vi "test Write and Read Signed Integer Array.vi"(8 "error in (no error)":errorcluster, 11 "TestCase in":refnum<class "Read Value Tests.lvclass">) -> (0 "error out":errorcluster, 3 "TestCase out":refnum<class "Read Value Tests.lvclass">)   [LabVIEW 2017, in "Mem Buff Tests.lvlib" / "Read Value Tests.lvclass"]
uses:
  Read Value Tests.lvclass
  Read Value Tests.lvclass/Read Value Tests.ctl
  Engine/Classes/Buffer/Read 1D I8.vi
  Engine/Classes/Buffer/Read 1D I16.vi
  Engine/Classes/Buffer/Read 1D I32.vi
  Engine/Classes/Buffer/Read 1D I64.vi
  <vilib>/addons/_JKI Toolkits/VI Tester/TestCase.llb/TestCase.lvclass
  Engine/Classes/Buffer/Buffer.lvclass
  C:/Program Files (x86)/National Instruments/LabVIEW 2017/vi.lib/addons/_JKI Toolkits/VI Tester/TestCase.llb/TestCase.lvclass
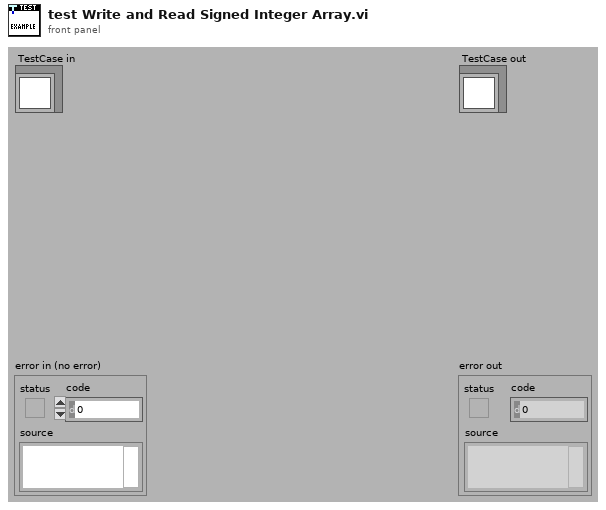
[diagram p1: front panel]
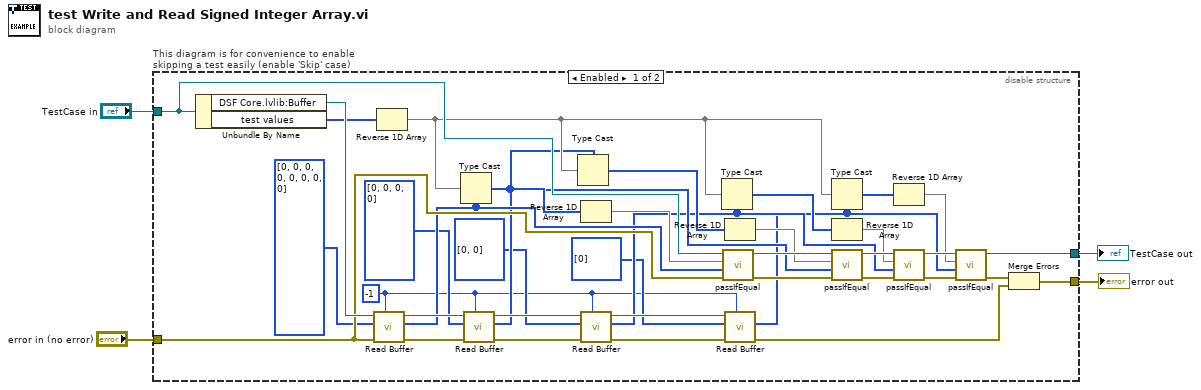
[diagram p0: block diagram]
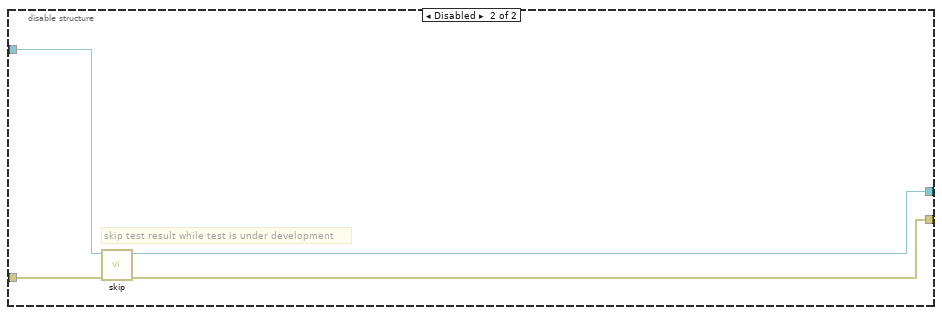
[diagram p2: hidden frame]
diagram:
  n1 = disable-structure "This diagram is for convenience to enable skipping a test easily (enable 'Skip' case)" shown="Enabled" {
    disable-tunnel: "TestCase in" -> [w24 w46]
    disable-tunnel: [w25 w44] -> w1
    disable-tunnel: [w21 w45] -> w2
    disable-tunnel: "error in (no error)" -> [w22 w43]
    frame Enabled {
      w5 = i64 -1 ("count")
      n2 = Unbundle By Name(w24) -> ("DSF Core.lvlib:Buffer"=w23:refnum<class "Buffer.lvclass">, "test values"=w19:u8[])
      n3 = call-poly "Read Buffer.vi"("count"=w5, "error in (no error)"=w22, "buffer in"=i8[] [0, 0, 0, 0, 0, 0, 0, 0], "Buffer in"=w23) -> ("error out"=w41:errorcluster, "buffer out"=w13:i8[], "Buffer out"=w42:refnum<class "Buffer.lvclass">)  [unwired: 4 in, 1 out]
      n4 = Reverse 1D Array(array=w19) -> (reversed array=w18:u8[])
      n5 = Type Cast(type=w13, x=w18) -> (*(type *) &x=w36:i8[])
      n6 = call-poly "Read Buffer.vi"("count"=w5, "error in (no error)"=w41, "buffer in"=i16[] [0, 0, 0, 0], "Buffer in"=w42) -> ("error out"=w39:errorcluster, "buffer out"=w10:i16[], "Buffer out"=w40:refnum<class "Buffer.lvclass">)  [unwired: 4 in, 1 out]
      n7 = Type Cast(type=w10, x=w18) -> (*(type *) &x=w35:i16[])
      n8 = Reverse 1D Array(array=w36) -> (reversed array=w17:i8[])
      n9 = call-poly "Read Buffer.vi"("count"=w5, "error in (no error)"=w39, "buffer in"=i32[] [0, 0], "Buffer in"=w40) -> ("error out"=w37:errorcluster, "buffer out"=w8:i32[], "Buffer out"=w38:refnum<class "Buffer.lvclass">)  [unwired: 4 in, 1 out]
      n10 = Type Cast(type=w8, x=w18) -> (*(type *) &x=w34:i32[])
      n11 = call-dynamic "passIfEqual.vi"("error in (no error)"=w22, "y"=w13, "x"=w17, "TestCase in"=w24) -> ("error out"=w29:errorcluster, "TestCase out"=w30:refnum<class "Read Value Tests.lvclass">)  [unwired: 6 in]
      n12 = Reverse 1D Array(array=w35) -> (reversed array=w16:i16[])
      n13 = call-poly "Read Buffer.vi"("count"=w5, "error in (no error)"=w37, "buffer in"=i64[] [0], "Buffer in"=w38) -> ("error out"=w20:errorcluster, "buffer out"=w6:i64[])  [unwired: 4 in, 2 out]
      n14 = Type Cast(type=w6, x=w18) -> (*(type *) &x=w33:i64[])
      n15 = Reverse 1D Array(array=w34) -> (reversed array=w15:i32[])
      n16 = call-dynamic "passIfEqual.vi"("error in (no error)"=w29, "y"=w10, "x"=w16, "TestCase in"=w30) -> ("error out"=w27:errorcluster, "TestCase out"=w28:refnum<class "Read Value Tests.lvclass">)  [unwired: 6 in]
      n17 = Reverse 1D Array(array=w33) -> (reversed array=w14:i64[])
      n18 = call-dynamic "passIfEqual.vi"("error in (no error)"=w27, "y"=w8, "x"=w15, "TestCase in"=w28) -> ("error out"=w32:errorcluster, "TestCase out"=w31:refnum<class "Read Value Tests.lvclass">)  [unwired: 6 in]
      n19 = call-dynamic "passIfEqual.vi"("error in (no error)"=w32, "y"=w6, "x"=w14, "TestCase in"=w31) -> ("error out"=w26:errorcluster, "TestCase out"=w25:refnum<class "Read Value Tests.lvclass">)  [unwired: 6 in]
      n20 = Merge Errors(w26, w20) -> (w21:errorcluster)
    }
    frame Disabled {
      # "skip test result while test is under development"
      n21 = call <vilib>:"skip.vi"("error in (no error)"=w43, "TestCase in"=w46) -> ("error out"=w45:errorcluster, "TestCase out"=w44:refnum<class "Read Value Tests.lvclass">)  [unwired: 8 in]
    }
  }
  "error out" <- w2
  "TestCase out" <- w1
